vi "Cleanup (User).vi"(8 "error in":errorcluster, 11 "Node in":refnum<class "AMS Cycler Template.lvclass">) -> (0 "error in":errorcluster, 3 "Node out":refnum<class "AMS Cycler Template.lvclass">)   [LabVIEW 2023, in "AMS Cycler Template.lvlib" / "AMS Cycler Template.lvclass"]
uses:
  AMS Cycler Template.lvclass
  AMS Cycler Template.lvclass/AMS Cycler Template.ctl
  Capabilities/Capabilities/High Level Capabilities/Cycler Cluster/Cycler Cluster.lvclass
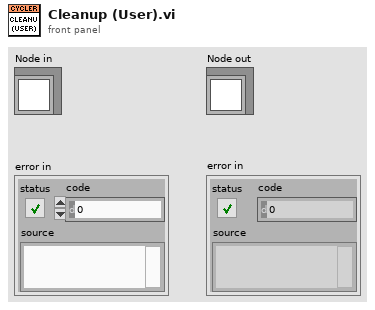
[diagram p1: front panel]
types:
  T1 = cluster{"OnOff.STS":i32, "Error.STS":i32, "Watchdog.STS":i32, "IsoMeasurement.STS":i32, "ParallelMode.STS":i32}
  T2 = cluster{"Error.STS":i32, "OutputEnable.STS":i32, "ControlMode.STS":u16, "Voltage.AV":dbl, "Current.AV":dbl, "Power.AV":dbl, "VoltageNominal.AV":dbl, "CurrentNominal.AV":dbl, "PowerNominal.AV":dbl, "ParameterSet.STS":i32}
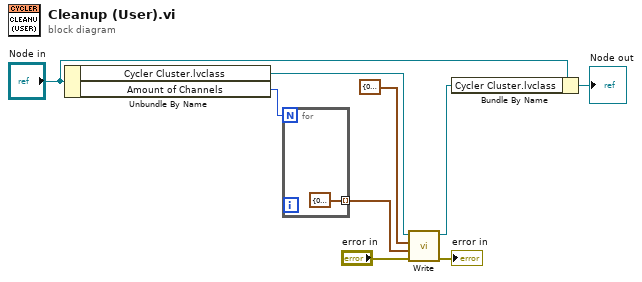
[diagram p0: block diagram]
diagram:
  n1 = Unbundle By Name("Node in") -> ("Cycler Cluster.lvclass"=w7:refnum<class "Cycler Cluster.lvclass">, "Amount of Channels"=w1:u32)
  n2 = for {
    N: w1 -> [_]
    tunnel: [T2 {"Error.STS"=0, "OutputEnable.STS"=0, "ControlMode.STS"=0, "Voltage.AV"=0.0, "Current.AV"=0.0, "Power.AV"=0.0, "VoltageNominal.AV"=0.0, "CurrentNominal.AV"=0.0, "PowerNominal.AV"=0.0, "ParameterSet.STS"=0} ("Producer Ch")] -> w2 mode=indexing
  }
  n3 = call "Write.vi"("error in"="error in", "Producer Ch"=w2, "Producer Control"=T1 {"OnOff.STS"=0, "Error.STS"=0, "Watchdog.STS"=0, "IsoMeasurement.STS"=0, "ParallelMode.STS"=0}, "Cycler Cluster.lvclass"=w7) -> ("error out"=→"error in":errorcluster, "output cluster"=w6:refnum<class "Cycler Cluster.lvclass">)  [unwired: 6 in]
  n4 = Bundle By Name(cluster="Node in", "Cycler Cluster.lvclass"=w6) -> (→"Node out":refnum<class "AMS Cycler Template.lvclass">)
